vi "Agilent SNA Restore.vi"(7 "Agilent SNA & SWP":T2, 8 "error in (no error)":errorcluster, 11 "VISA Resource Names":T1) -> (0 "error out":errorcluster {"code" format="%.0x"}, 3 "dup VISA Resource Names":T1)   [LabVIEW 2011]
uses:
  TypeDefs/Agilent SNA VISA.ctl
  TypeDefs/Agilent SNA Instrument Info.ctl
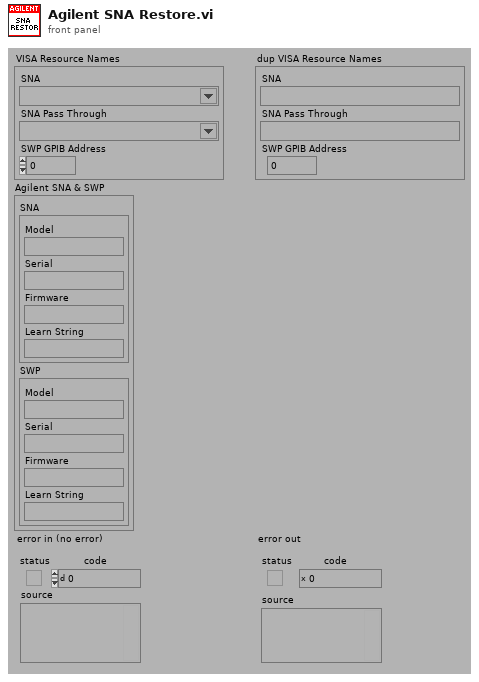
[diagram p1: front panel]
types:
  T1 = typedef "Agilent SNA VISA.ctl" = cluster{"SNA":refnum<visa-resource-name>, "SNA Pass Through":refnum<visa-resource-name>, "SWP GPIB Address":i32}
  T2 = typedef "Agilent SNA Instrument Info.ctl" = cluster{"SNA":cluster{"Model":string, "Serial":string, "Firmware":string, "Learn String":string}, "SWP":cluster{"Model":string, "Serial":string, "Firmware":string, "Learn String":string}}
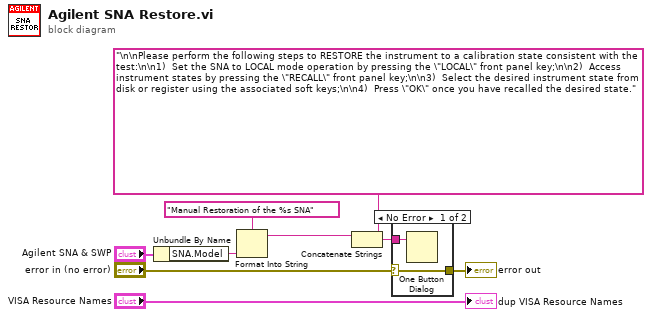
[diagram p0: block diagram]
diagram:
  n1 = Unbundle By Name("Agilent SNA & SWP") -> ("SNA.Model"=w7:string)
  n2 = Format Into String(format string="Manual Restoration of the %s SNA", w7) -> (resulting string=w6:string)  [unwired: 2 in, 1 out]
  n3 = Concatenate Strings(w6, "\n\nPlease perform the following steps to RESTORE the instrument to a calibration state consistent with the test:\n\n1)  Set the SNA to LOCAL mode operation by pressing the \"LOCAL\" front panel key;\n\n2)  Access instrument states by pressing the \"RECALL\" front panel key;\n\n3)  Select the desired instrument state from disk or register using the associated soft keys;\n\n4)  Press \"OK\" once you have recalled the desired state.") -> (w4:string)
  n4 = case shown="No Error" "error in (no error)" {
    selector: "error in (no error)" -> [w10 w12]
    tunnel: w4 -> [w11 _]
    tunnel: [w10 w12] -> w2
    frame No Error {
      n5 = One Button Dialog(message=w11) -> ()  [unwired: 2 out]
    }
    frame Error {
    }
  }
  "error out" <- w2
  "dup VISA Resource Names" <- "VISA Resource Names"
